vi "load_external_coordinates_MD.vi"() -> ()   [LabVIEW 2012]
uses:
  GFG/GFGDisplayRefsGet.vi
  <vilib>/Utility/file.llb/Read From Spreadsheet File (DBL).vi
  GFG/GFG library.lvlib
panel:
  out "error out":errorcluster
  in  "error in (no error)":errorcluster
  in  "stop":bool
  in  "file path (dialog if empty)":path
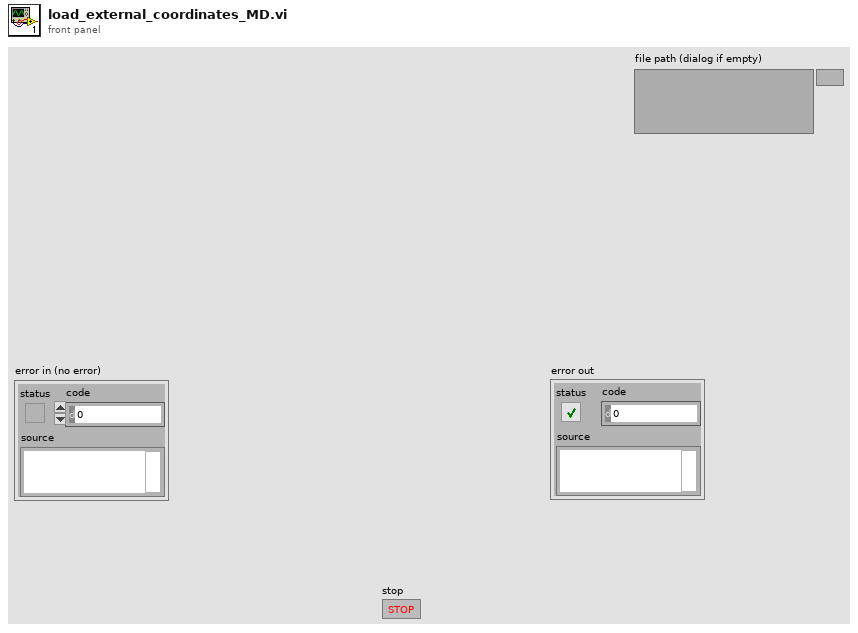
[diagram p1: front panel]
types:
  T1 = cluster{"Channel 1 small":refnum<vi>, "Channel 2 small":refnum<vi>, "Channel 3 small":refnum<vi>, "Channel 4 small":refnum<vi>, "Channel 1 large":refnum<vi>, "Channel 2 large":refnum<vi>, "Channel 3 large":refnum<vi>, "Channel 4 large":refnum<vi>, "RGB overlay":refnum<vi>, "ROI Image display":refnum<vi>, "arb line scan display":refnum<vi>, "Channel 5 large":refnum<vi>}
  T2 = cluster{"Contour Type":u32, "ROI Type":u32, i32[]}
  T3 = cluster{"Contour Type":u32, "ROI Type":u32, i32[]}[]
  T4 = cluster{i32[], cluster{"Contour Type":u32, "ROI Type":u32, i32[]}[]}
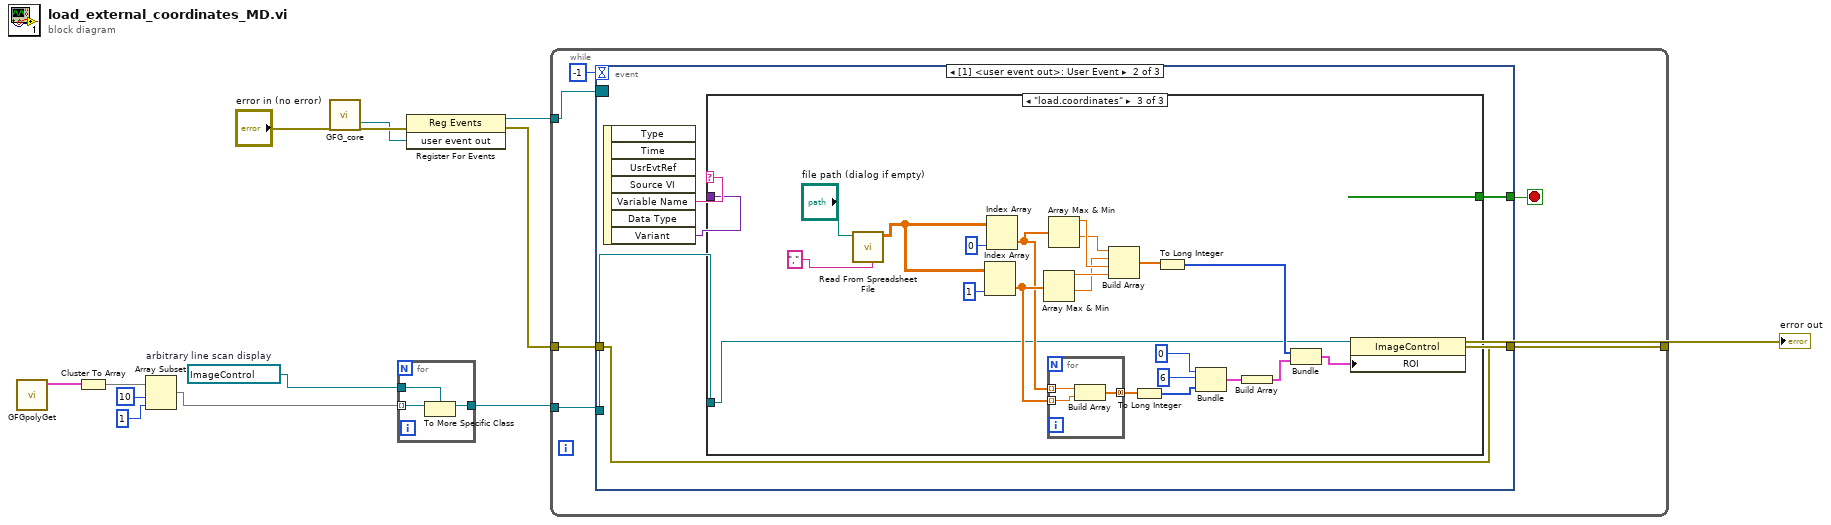
[diagram p0: block diagram]
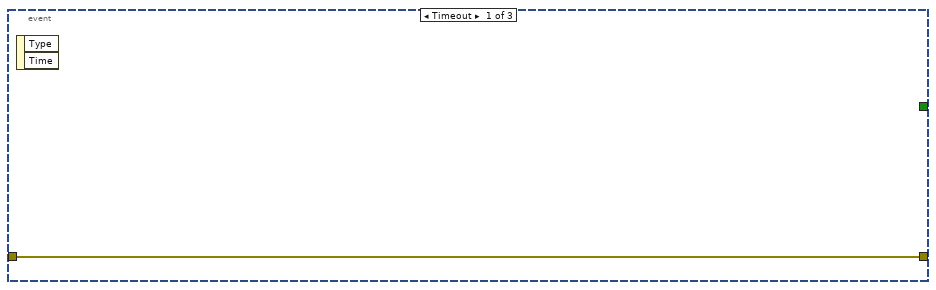
[diagram p2: hidden frame]
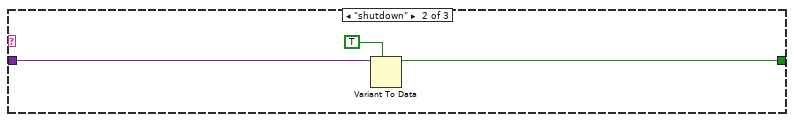
[diagram p4: hidden frame]
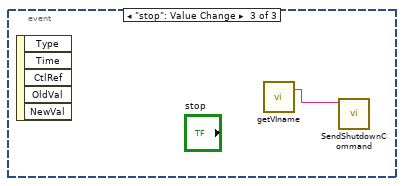
[diagram p5: hidden frame]
diagram:
  w9 = refnum<vi> refnum  # arbitrary line scan display
  n1 = call-poly "GFGpolyGet.vi"() -> ("DisplayRefsOut(generic class)"=w8:T1)  [unwired: 10 in, 1 out]
  n2 = Cluster To Array(cluster=w8) -> (array=w11:refnum<vi>[])
  n3 = Array Subset(array=w11, index=10, length=1) -> (w10:refnum<vi>[])
  n4 = call "GFG_core.vi"("error in (no error)"="error in (no error)") -> ("user event out"=w3:refnum<user-event>, "error out"=w4:errorcluster)  [unwired: 12 in, 5 out]
  n5 = for {
    tunnel: w10 -> [w16] mode=indexing
    tunnel: w9 -> [w15]
    tunnel: [w14] -> w1
    n6 = To More Specific Class(target class=w15, reference=w16) -> (specific class reference=w14:refnum<vi>)  [unwired: 1 in, 1 out]
  }
  n7 = register-events(error in=w4, w3) -> (reference out=w2:refnum<event-registration>, error out=w6:errorcluster)  [unwired: 1 in]
  n8 = while {
    tunnel: w2 -> [w22]
    tunnel: w6 -> [w20]
    tunnel: [w19] -> w7
    tunnel: w1 -> [w17]
    stop <- w21 stop-if-true
    n9 = event shown="[1] <user event out>: User Event" {
      selector: w22 -> [_ _ _]
      dyn-events: _ -> [_ _ _]
      timeout: -1 -> [_ _ _]
      tunnel: [_ w26 _] -> w21
      tunnel: w20 -> [w23 w25 _]
      tunnel: [w23 w25 _] -> w19
      tunnel: w17 -> [_ w24 _]
      event Timeout {
        n10 = event-data() -> ()  [unwired: 1 in, 2 out]
      }
      event User Event {
        n11 = event-data() -> ("Variable Name"=w28:string, "Variant"=w27:variant)  [unwired: 1 in, 5 out]
        n12 = case shown="\"load.coordinates\"" w28 {
          tunnel: w27 -> [_ w31 _]
          tunnel: [_ w29 _] -> w26
          tunnel: w24 -> [_ _ w32]
          frame "False", Default {
          }
          frame "shutdown" {
            n13 = Variant To Data(type=TRUE ("want seconds? (F)"), Variant=w31) -> (data=w29:bool)  [unwired: 1 in, 1 out]
          }
          frame "load.coordinates" {
            n14 = call-poly <vilib>:"Read From Spreadsheet File.vi"("delimiter (\\t)"="," ("delimiter (\\t)"), "file path (dialog if empty)"="file path (dialog if empty)") -> ("all rows"=w37:dbl[][])  [unwired: 5 in, 4 out]
            n15 = Index Array(array=w37, index (col)=1 ("disabled index (col)")) -> (element=w45:dbl[])  [unwired: 1 in]
            n16 = Index Array(array=w37, index (col)=0 ("disabled index (col)")) -> (element=w44:dbl[])  [unwired: 1 in]
            n17 = Array Max & Min(array=w45) -> (max value=w42:dbl, min value=w40:dbl)  [unwired: 2 out]
            n18 = for {
              tunnel: w44 -> [w55] mode=indexing
              tunnel: w45 -> [w54] mode=indexing
              tunnel: [w53] -> w48 mode=concatenating
              n19 = Build Array(w55, w54) -> (w53:dbl[])
            }
            n20 = Array Max & Min(array=w44) -> (max value=w41:dbl, min value=w39:dbl)  [unwired: 2 out]
            n21 = Build Array(w39, w40, w41, w42) -> (w43:dbl[])
            n22 = To Long Integer(number=w48) -> (32bit integer=w49:i32[])
            n23 = To Long Integer(number=w43) -> (32bit integer=w52:i32[])
            n24 = Bundle("Contour Type"=u32 0, "ROI Type"=u32 6, w49) -> (w50:T2)  [unwired: 1 in]
            n25 = Build Array(w50) -> (w51:T3)
            n26 = Bundle(w52, w51) -> (w34:T4)  [unwired: 1 in]
            n27 = property class="ImageControl"(reference=w32, "ROI"=w34) -> ()  [unwired: 1 in, 2 out]
          }
        }
      }
      event "stop": Value Change {
        n28 = event-data() -> ()  [unwired: 1 in, 5 out]
        n29 = call "getVIname.vi"() -> ("VI name"=w56:string)  [unwired: 19 in]
        n30 = call "SendShutdownCommand.vi"("Source VI"=w56) -> ()  [unwired: 11 in]
      }
    }
  }
  "error out" <- w7
